vi "Test_LogValueEvent_LogMultipleDBL_MatchFormattoString.vi"(8 "error in (no error)":errorcluster, 11 "TestCase in":refnum<class "TestLogValue.lvclass">) -> (0 "error out":errorcluster, 3 "TestCase out":refnum<class "TestLogValue.lvclass">)   [LabVIEW 2019, in "TestLogValue.lvclass"]
uses:
  TestLogValue.lvclass
  Source/Composed Log/Types/Log Level.ctl
  Source/Composed Log/LoggerReference/LoggerReference.lvclass/LoggerReference.ctl
  Source/LVQueue Sink/LVQueue Sink.lvclass/LVQueue Sink.ctl
  272d61b2-f49c-486c-9daf-337ffb054b40.vi
  154dbc8a-62f5-4aa1-ad82-2a3c469f95b7.vi
  Source/Composed Log/LoggerReference/Return Aggregate Queues.vi
  Source/Composed Log/LoggerReference/Add Aggregate Log.vi
  272d61b2-f49c-486c-9daf-337ffb054b40.vi/ca34ee31-fc47-4f65-ade2-e0d33578437a.vi
  154dbc8a-62f5-4aa1-ad82-2a3c469f95b7.vi/b9763440-381f-4620-8ec2-275a2cbfe1d8.vi
  Source/Composed Log/LoggerReference/Get Formatter.vi
  Source/Composed Log/LoggerReference/Get Valid Event Time.vi
  Source/Composed Log/LoggerReference/Log Event.vi
  Source/Composed Log/LoggerReference/Send Add Sink.vi
  Source/Composed Log/LoggerReference/Log.vi
  Source/Composed Log/LoggerReference/Remove Stale Logs.vi
  Source/LVQueue Sink/LVQueue Sink.lvclass
  C:/CS/Log/Source/Composed Log/Log Sink/Log Sink.lvclass
  Source/Composed Log/Application Logger/Launch Worker Loop.vi
  Source/Composed Log/LoggerReference/Initialize Logger Instance.vi
  Source/Composed Log/LoggerReference/LoggerReference.lvclass
  Source/Composed Log/IErrorFormat/IErrorFormat.lvclass
  Source/Composed Log/Log Sink/Log Sink.lvclass
  <vilib>/addons/_JKI Toolkits/VI Tester/TestCase.llb/TestCase.lvclass
  Source/Composed Log/Composed Log.lvlib
  C:/Program Files (x86)/National Instruments/LabVIEW 2019/vi.lib/addons/_JKI Toolkits/VI Tester/TestCase.llb/TestCase.lvclass
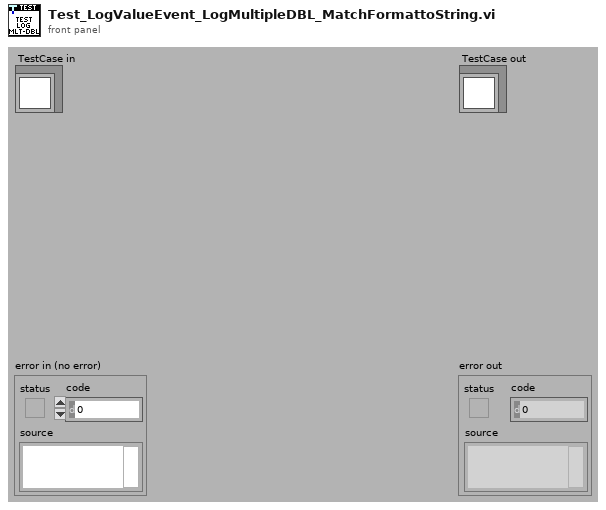
[diagram p1: front panel]
types:
  T1 = typedef "Composed Log.lvlib/Log Level.ctl" = enum16{"Debug", "Info", "Warning", "Error", "Critical"}
  T2 = typedef "Composed Log.lvlib/Log Packet.ctl" = cluster{"Data To Log":string, "Source":string, "Event Level":T1, "Event Time":timestamp}
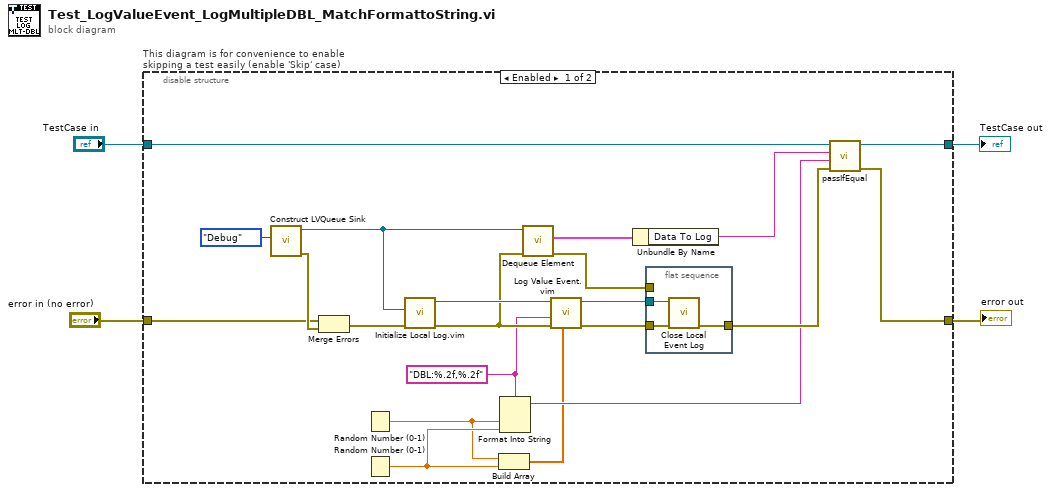
[diagram p0: block diagram]
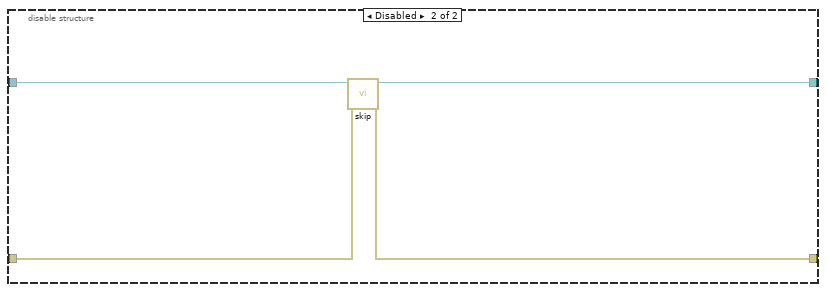
[diagram p2: hidden frame]
diagram:
  n1 = disable-structure "This diagram is for convenience to enable skipping a test easily (enable 'Skip' case)" shown="Enabled" {
    disable-tunnel: "TestCase in" -> [w19 w32]
    disable-tunnel: [w18 w30] -> w1
    disable-tunnel: [w16 w31] -> w3
    disable-tunnel: "error in (no error)" -> [w17 w29]
    frame Enabled {
      w11 = "DBL:%.2f,%.2f" ("Data To Log")
      n2 = call "Construct LVQueue Sink.vi"("LogLevel"=Log_Level."Debug") -> ("error out"=w22:errorcluster, "LVQueue Sink out"=w20:refnum<class "LVQueue Sink.lvclass">)  [unwired: 9 in]
      n3 = Merge Errors(w17, w22) -> (w21:errorcluster)
      n4 = Random Number (0-1)() -> (number: 0 to 1=w6:dbl)
      n5 = Random Number (0-1)() -> (number: 0 to 1=w7:dbl)
      n6 = call "Initialize Local Log.vim"("error in (no error)"=w21, "Startup Sink(s)"=w20) -> ("error out"=w14:errorcluster, "Log Instance Reference"=w15:refnum<class "LoggerReference.lvclass">)  [unwired: 7 in, 1 out]
      n7 = Build Array(w6, w7) -> (w5:dbl[])
      n8 = Format Into String(format string=w11, w6, w7) -> (resulting string=w9:string)  [unwired: 2 in, 1 out]
      n9 = call "Dequeue Element.vi"("error in (no error)"=w14, "LVQueue Sink in"=w20) -> ("error out"=w25:errorcluster, "Log Packet"=w23:T2)  [unwired: 6 in, 2 out]
      n10 = call "Log Value Event.vim"("Value(s)"=w5, "error in (no error)"=w14, "Log Message Format String"=w11, "LoggerReference in"=w15) -> ("error out"=w13:errorcluster, "LoggerReference out"=w12:refnum<class "LoggerReference.lvclass">)  [unwired: 6 in]
      n11 = Unbundle By Name(w23) -> ("Data To Log"=w10:string)
      n12 = flat-sequence {
        tunnel: [w27] -> w24
        tunnel: w13 -> [w28]
        tunnel: w25 -> [_]
        tunnel: w12 -> [w26]
        frame #0 {
          n13 = call "Close Local Event Log.vi"("error in (no error)"=w28, "Log Instance"=w26) -> ("error out"=w27:errorcluster)  [unwired: 9 in]
        }
      }
      n14 = call-dynamic "passIfEqual.vi"("error in (no error)"=w24, "y"=w9, "x"=w10, "TestCase in"=w19) -> ("error out"=w16:errorcluster, "TestCase out"=w18:refnum<class "TestLogValue.lvclass">)  [unwired: 6 in]
    }
    frame Disabled {
      # "skip test result while test is under development"
      n15 = call <vilib>:"skip.vi"("error in (no error)"=w29, "TestCase in"=w32) -> ("error out"=w31:errorcluster, "TestCase out"=w30:refnum<class "TestLogValue.lvclass">)  [unwired: 8 in]
    }
  }
  "error out" <- w3
  "TestCase out" <- w1
